vi "Format SQL CREATE TABLE.vi"(8 "error in (no error)":errorcluster, 10 "Data (Dictionary)":T1[](array[typedef]), 11 "Table name":string="my table") -> (0 "error out":errorcluster, 2 "SQL":string="BEGIN;\nCREATE TABLE my table (\n  test_id Serial PRIMARY KEY,\n  key1 double precision,\n\t\tkey2 double precision);\nCOMMIT;")   [LabVIEW 2019, in "Data.PG.lvclass"]
uses:
  Data.PG.lvclass
  <vilib>/Utility/Data Type/NI_Data Type.lvlib
  Data/Data.lvclass
  Data/Typedefs/Dictionary--cluster.ctl
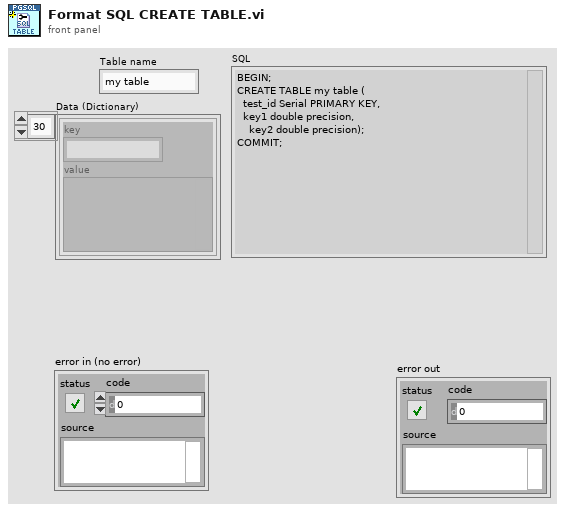
[diagram p1: front panel]
types:
  T1 = typedef "Data.lvclass/Dictionary--cluster.ctl" = cluster{"key":string, "value":variant}
  T2 = typedef "NI_Data Type.lvlib/Data Type.ctl" = enum8{"Invalid Type", "Void", "I8", "I16", "I32", "I64", "U8", "U16", "U32", "U64", "Single Float", "Double Float", "Extended Float", "Single Complex", "Double Complex", "Extended Complex", "Enum U8", "Enum U16", "Enum U32", "Enum U64", "Single Float With Unit", "Double Float With Unit", "Extended Float With Unit", "Single Complex with Unit", "Double Complex with Unit", "Extended Complex with Unit", "Boolean", "String", "Path", "Picture", "Tag", "Array", "Cluster", "Variant", "LV Variant", "Waveform", "Timestamp", "Digital Waveform", "Digital Data", "ExpressData", "Refnum", "External Data", "VI", "Poly VI", "LabVIEW Class Instance", "Fixed Point", "Set Collection", "Map Collection"}
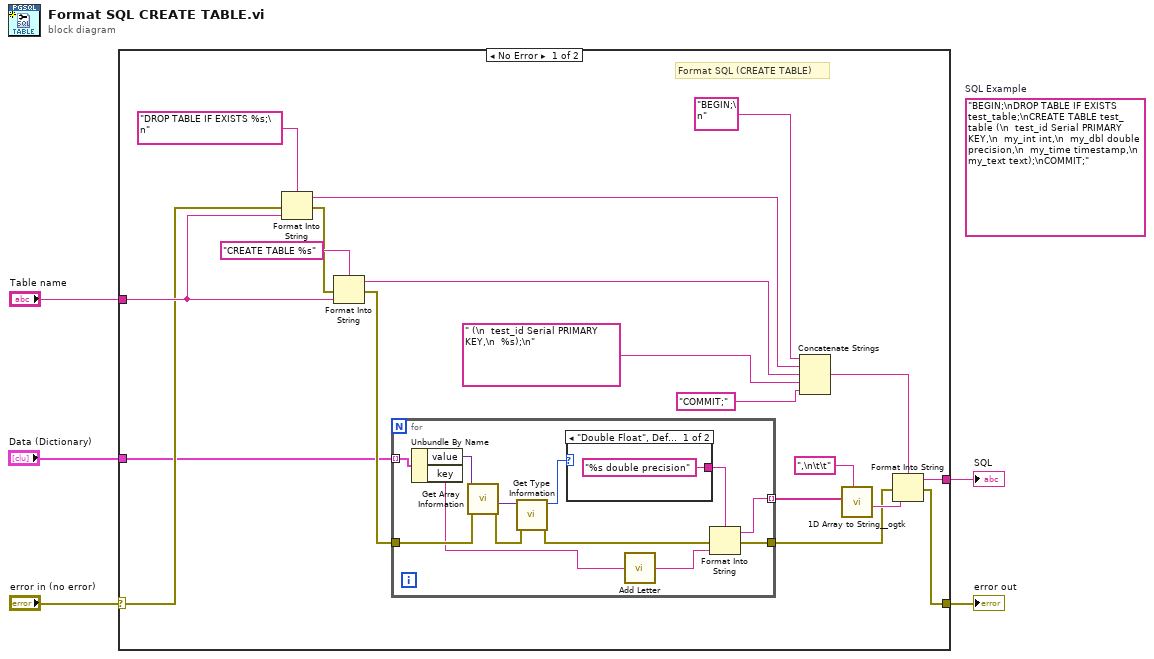
[diagram p0: block diagram]
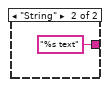
[diagram p2: hidden frame]
diagram:
  (unwired) "BEGIN;\nDROP TABLE IF EXISTS test_table;\nCREATE TABLE test_table (\n  test_id Serial PRIMARY KEY,\n  my_int int,\n  my_dbl double precision,\n  my_time timestamp,\n  my_text text);\nCOMMIT;"  # SQL Example
  n1 = case shown="No Error" "error in (no error)" {
    selector: "error in (no error)" -> [w9 w39]
    tunnel: [w24 _] -> w5
    tunnel: [w23 w39] -> w4
    tunnel: "Table name" -> [w13 _]
    tunnel: "Data (Dictionary)" -> [w8 _]
    frame No Error {
      # "Format SQL (CREATE TABLE)"
      n2 = Format Into String(format string="DROP TABLE IF EXISTS %s;\n" ("SQL"), error in=w9, w13) -> (resulting string=w7:string, error out=w12:errorcluster)  [unwired: 1 in]
      n3 = Format Into String(format string="CREATE TABLE %s" ("SQL"), error in=w12, w13) -> (resulting string=w17:string, error out=w18:errorcluster)  [unwired: 1 in]
      n4 = for {
        tunnel: [w36] -> w22 mode=indexing
        tunnel: w18 -> [w32]
        tunnel: [w35] -> w20
        tunnel: w8 -> [w34] mode=indexing
        n5 = Unbundle By Name(w34) -> ("value"=w27:variant, "key"=w26:string)
        n6 = call <vilib>:"Get Array Information.vi"("error in (no error)"=w32, "variant"=w27) -> ("error out"=w31:errorcluster, "array element data type"=w33:variant)  [unwired: 6 in, 2 out]
        n7 = call <vilib>:"Get Type Information.vi"("error in (no error)"=w31, "variant"=w33) -> ("error out"=w30:errorcluster, "type"=w28:T2)  [unwired: 5 in, 3 out]
        n8 = case shown="\"Double Float\", Default" w28 {
          tunnel: ["%s double precision" ("format string") "%s text" ("format string")] -> w29
          frame "Double Float", Default {
          }
          frame "String" {
          }
        }
        n9 = call "Add Letter.vi"("string"=w26) -> ("result string"=w25:string)
        n10 = Format Into String(format string=w29, error in=w30, w25) -> (resulting string=w36:string, error out=w35:errorcluster)  [unwired: 1 in]
      }
      n11 = Concatenate Strings("BEGIN;\n" ("SQL"), w7, w17, " (\n  test_id Serial PRIMARY KEY,\n  %s);\n" ("SQL"), "COMMIT;" ("SQL")) -> (w19:string)
      n12 = call <userlib>:"1D Array to String__ogtk.vi"("delimiter (Tab)"=",\n\t\t", "Array of Strings"=w22) -> ("delimited string"=w21:string)  [unwired: 9 in]
      n13 = Format Into String(format string=w19, error in=w20, w21) -> (resulting string=w24:string, error out=w23:errorcluster)  [unwired: 1 in]
    }
    frame Error {
    }
  }
  "SQL" <- w5
  "error out" <- w4
